vi "getHWCStatus.vi"(8 "error in (no error)":errorcluster, 10 "status in":refnum<vi>, 11 "ExperimentRunner in":refnum<class "ExperimentRunner.lvclass">) -> (0 "error out":errorcluster, 1 "status":T1(ring), 2 "status out":refnum<vi>, 3 "ExperimentRunner out":refnum<class "ExperimentRunner.lvclass">)   [LabVIEW 2009, in "Views.lvlib" / "ExperimentControl.lvlib" / "ExperimentRunner.lvclass"]
uses:
  ExperimentRunner.lvclass
  ExperimentRunner.lvclass/ExperimentRunner.ctl
  Hal/HWController/HWControllerEvents/HWControllerEvents.lvclass
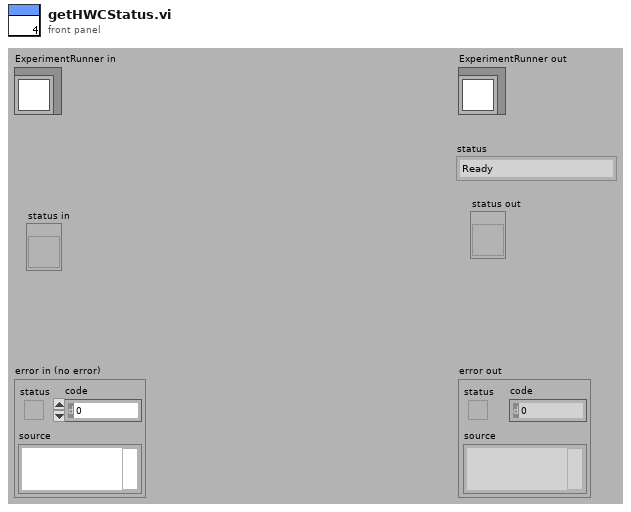
[diagram p1: front panel]
types:
  T1 = enum16{"Ready", "Compiling", "Configured", "Running", "Stopping", "Unresolved Error"}
  T2 = enum16{"start", "stop", "statusInquiry", "configure", "resetError", "resourcesInquiry", "reserveResources", "initialise", "resetAllChannels", "staticUpdate", "close", "HWStatus", "error", "resourcesAvailable", "resourcesReserved", "compilerError", "compiledScript", "compilingScript", "runScript", "configureCompiledScript"}
  T3 = cluster{"incomingEventTypes":cluster{"start":cluster{"Boolean":bool}, "stop":cluster{"Boolean":bool}, "statusInquiry":cluster{"Boolean":bool}, "configure":cluster{"DPScriptPath":path, "TimeStamp":string, "HWLoop?":bool}, "resetError":cluster{"Boolean":bool}, "resourcesInquiry":cluster{"Boolean":bool}, "reserveResources":cluster{"HWList":string[]}, "initialise":cluster{"HWList":string[]}, "close":cluster{"Boolean":bool}, "resetAllChannels":cluster{"Boolean":bool}, "staticChannelUpdate":cluster{"channel_address":string, "calibratedValue":dbl}, "runScript":cluster{"DPScriptPath":path, "TimeStamp":string, "HWLoop?":bool}, "compilingScript":cluster{"Path":path}, "compiledScript":cluster{"Path":path, "timeCompileAt":string}, "compilerError":cluster{"Path":path}, "configureCompiledScript":cluster{"DPScriptPath":path, "TimeStamp":string, "HWLoop?":bool, "CompiledScript":cluster{"ScriptListCompiler.lvclass":refnum<class "ScriptListCompiler.lvclass">, "aoChannels":refnum<class "AnalogOutput.lvclass">[], "doChannels":refnum<class "DigitalOutput.lvclass">[], "rfChannels":refnum<class "DDSOutput.lvclass">[]}}, "restartCompiler":cluster{"restart":bool}, "staticRfChannelUpdate":cluster{"channel_address":string, "Output":cluster{"Frequency(MHz)":dbl, "Amplitude":dbl, "Phase":dbl, "OutputForm":enum16{"Sine", "Square", "Triangle", "Arbitrary"}}}}, "outgoingEventTypes":cluster{"HWStatus":cluster{"status":enum16{"Ready", "Compiling", "Configured", "Running", "Stopping", "Unresolved Error"}}, "error":cluster{"error out":errorcluster}, "resourcesAvailable":cluster{"availableHWList":string[], "reservedHWList":string[]}, "resourcesReserved":cluster{"reservedHWList":string[]}}}
  T4 = cluster{"status":enum16{"Ready", "Compiling", "Configured", "Running", "Stopping", "Unresolved Error"}}
  T5 = cluster{"eventId":enum16{"start", "stop", "statusInquiry", "configure", "resetError", "resourcesInquiry", "reserveResources", "initialise", "resetAllChannels", "staticUpdate", "close", "HWStatus", "error", "resourcesAvailable", "resourcesReserved", "compilerError", "compiledScript", "compilingScript", "runScript", "configureCompiledScript"}, "statusInquiry":cluster{"Boolean":bool}}
  T6 = enum16{"start", "stop", "statusInquiry", "configure", "resetError", "resourcesInquiry", "reserveResources", "initialise", "resetAllChannels", "staticUpdate", "close", "HWStatus", "error", "resourcesAvailable", "resourcesReserved", "compilerError", "compiledScript", "compilingScript", "runScript", "configureCompiledScript", "restartCompiler", "staticRfChannelUpdate"}
  T7 = cluster{"eventId":enum16{"start", "stop", "statusInquiry", "configure", "resetError", "resourcesInquiry", "reserveResources", "initialise", "resetAllChannels", "staticUpdate", "close", "HWStatus", "error", "resourcesAvailable", "resourcesReserved", "compilerError", "compiledScript", "compilingScript", "runScript", "configureCompiledScript"}, bool}
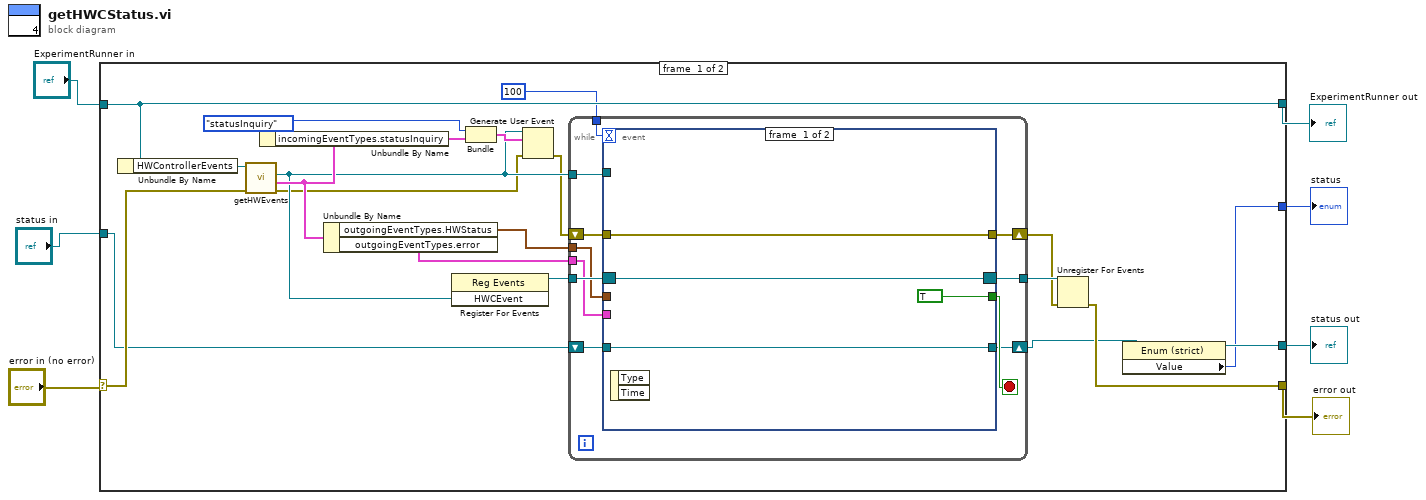
[diagram p0: block diagram]
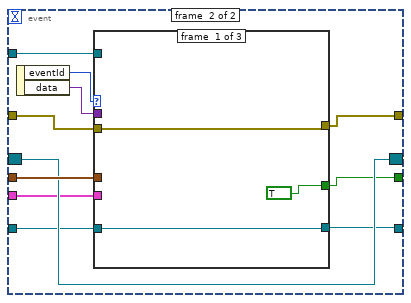
[diagram p2: hidden frame]
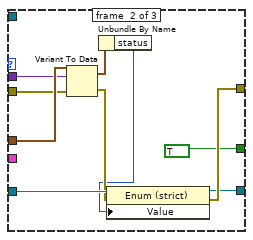
[diagram p3: hidden frame]
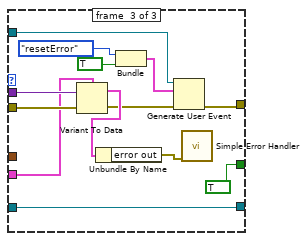
[diagram p4: hidden frame]
diagram:
  n1 = case shown="No Error" "error in (no error)" {
    selector: "error in (no error)" -> [w26 w83]
    tunnel: [w21 w83] -> w6
    tunnel: [w28 w82] -> w4
    tunnel: "ExperimentRunner in" -> [w28 w82]
    tunnel: [w8 _] -> w3
    tunnel: "status in" -> [w19 w81]
    tunnel: [w9 w81] -> w1
    frame #0 {
      n2 = Unbundle By Name(w28) -> ("HWControllerEvents"=w27:refnum<class "HWControllerEvents.lvclass">)
      n3 = call-dynamic "getHWEvents.vi"("error in (no error)"=w26, "HWControllerEvents in"=w27) -> ("error out"=w14:errorcluster, "eventDataTypes"=w18:T3, "HWCEvent"=w15:refnum<user-event>)  [unwired: 6 in, 1 out]
      n4 = Unbundle By Name(w18) -> ("incomingEventTypes.statusInquiry"=w17:cluster{"Boolean":bool})
      n5 = Unbundle By Name(w18) -> ("outgoingEventTypes.HWStatus"=w24:T4, "outgoingEventTypes.error"=w20:cluster{"error out":errorcluster})
      n6 = register-events(w15) -> (reference out=w25:refnum<event-registration>)  [unwired: 2 in, 1 out]
      n7 = Bundle("eventId"=T2."statusInquiry", "statusInquiry"=w17) -> (w16:T5)  [unwired: 1 in]
      n8 = Generate User Event(user event=w15, event data cluster=w16, error in=w14) -> (error out=w13:errorcluster)  [unwired: 1 out]
      n9 = while {
        tunnel: w25 -> [w39]
        tunnel: w24 -> [w38]
        shift-right: [w36] -> w22
        shift-left: w13 -> [w37]
        tunnel: [w35] -> w23
        tunnel: w20 -> [w33]
        tunnel: w15 -> [w32]
        shift-right: [w30] -> w10
        shift-left: w19 -> [w31]
        tunnel: 100 -> [w29]
        stop <- w34 stop-if-true
        n10 = event shown="[1] <HWCEvent>: User Event" {
          selector: w39 -> [w41 w51]
          dyn-events: [w41 w51] -> w35
          timeout: w29 -> [_ _]
          tunnel: w38 -> [_ w52]
          tunnel: w37 -> [w40 w50]
          tunnel: [w40 w49] -> w36
          tunnel: [TRUE w48] -> w34
          tunnel: w33 -> [_ w47]
          tunnel: w32 -> [_ w46]
          tunnel: w31 -> [w43 w45]
          tunnel: [w43 w44] -> w30
          event #0 {
            n11 = event-data() -> ()  [unwired: 1 in, 2 out]
          }
          event #1 {
            n12 = event-data() -> ("eventId"=w54:T6, "data"=w53:variant)  [unwired: 1 in]
            n13 = case shown="\"HWStatus\"" w54 {
              tunnel: w53 -> [_ w66 w80]
              tunnel: w52 -> [_ w67 _]
              tunnel: w50 -> [w57 w65 w79]
              tunnel: [w57 w61 w73] -> w49
              tunnel: [TRUE TRUE TRUE] -> w48
              tunnel: w47 -> [_ _ w77]
              tunnel: w46 -> [_ _ w72]
              tunnel: w45 -> [w56 w63 w69]
              tunnel: [w56 w60 w69] -> w44
              frame #0 {
              }
              frame #1 {
                n14 = Variant To Data(error in=w65, Variant=w66, type=w67) -> (error out=w62:errorcluster, data=w64:T4)
                n15 = Unbundle By Name(w64) -> ("status"=w58:T1)
                n16 = property class="Enum (strict)"(reference=w63, error in=w62, "Value"=w58) -> (reference out=w60:refnum<vi>, error out=w61:errorcluster)
              }
              frame #2 {
                n17 = Variant To Data(error in=w79, Variant=w80, type=w77) -> (error out=w74:errorcluster, data=w76:cluster{"error out":errorcluster})
                n18 = Unbundle By Name(w76) -> ("error out"=w75:errorcluster)
                n19 = Bundle("eventId"=T2."resetError", TRUE) -> (w70:T7)  [unwired: 1 in]
                n20 = Generate User Event(user event=w72, event data cluster=w70, error in=w74) -> (error out=w73:errorcluster)  [unwired: 1 out]
                n21 = call <vilib>:"Simple Error Handler.vi"("error in (no error)"=w75) -> ()  [unwired: 4 in, 5 out]
              }
            }
          }
        }
      }
      n22 = Unregister For Events(event registration refnum=w23, error in=w22) -> (error out=w21:errorcluster)
      n23 = property class="Enum (strict)"(reference=w10) -> (reference out=w9:refnum<vi>, "Value"=w8:T1)  [unwired: 1 in, 1 out]
    }
    frame #1 {
    }
  }
  "error out" <- w6
  "ExperimentRunner out" <- w4
  "status" <- w3
  "status out" <- w1
